vi "2 (1).vi"() -> ()   [LabVIEW 2015]
uses:
  <vilib>/NXT/Block Support/NXT_InputPort.ctl
  <vilib>/NXT/Block Support/NXT_OutputPort.ctl
  <vilib>/NXT/Dual Mode Library/Sensors/Sonar_cm.vi
  <vilib>/NXT/NXTIO Xnodes/NXTIONodeSubVIs/NXTMoveMotors.vi
  <vilib>/NXT/Dual Mode Library/Waits/Wait_Num.vi
  <vilib>/NXT/NXTIO Xnodes/AddressXNode/NXTIOAddress.xnode
  <vilib>/NXT/Subs/LVHSConnector.ctl
  <vilib>/NXT/NXTIO Xnodes/NXTIOXNode/NXTIO.xnode
  <vilib>/NXT/LegoClasses/BrickReference/BrickReference.lvclass
panel:
  in  "Power/Speed 4":i8=75
  in  "Power/Speed 3":i8=75
  in  "Time (1 sec) 2":sgl=1.0
  in  "Time (1 sec)":sgl=1.0
  in  "Power/Speed 1":i8=75
  in  "Port (Port 4)":T1=3 items=["Port 1", "Port 2", "Port 3", "Port 4"]
  in  "stop":bool
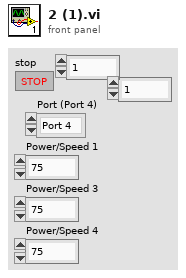
[diagram p1: front panel]
types:
  T1 = typedef "NXT_InputPort.ctl" = u32
  T2 = typedef "NXT_OutputPort.ctl" = u8
  T3 = cluster{"Output Port":T2, "Output Port 2":T2, "Output Port 3":T2}
  T4 = typedef "LVHSConnector.ctl" = refnum<class "BrickReference.lvclass">
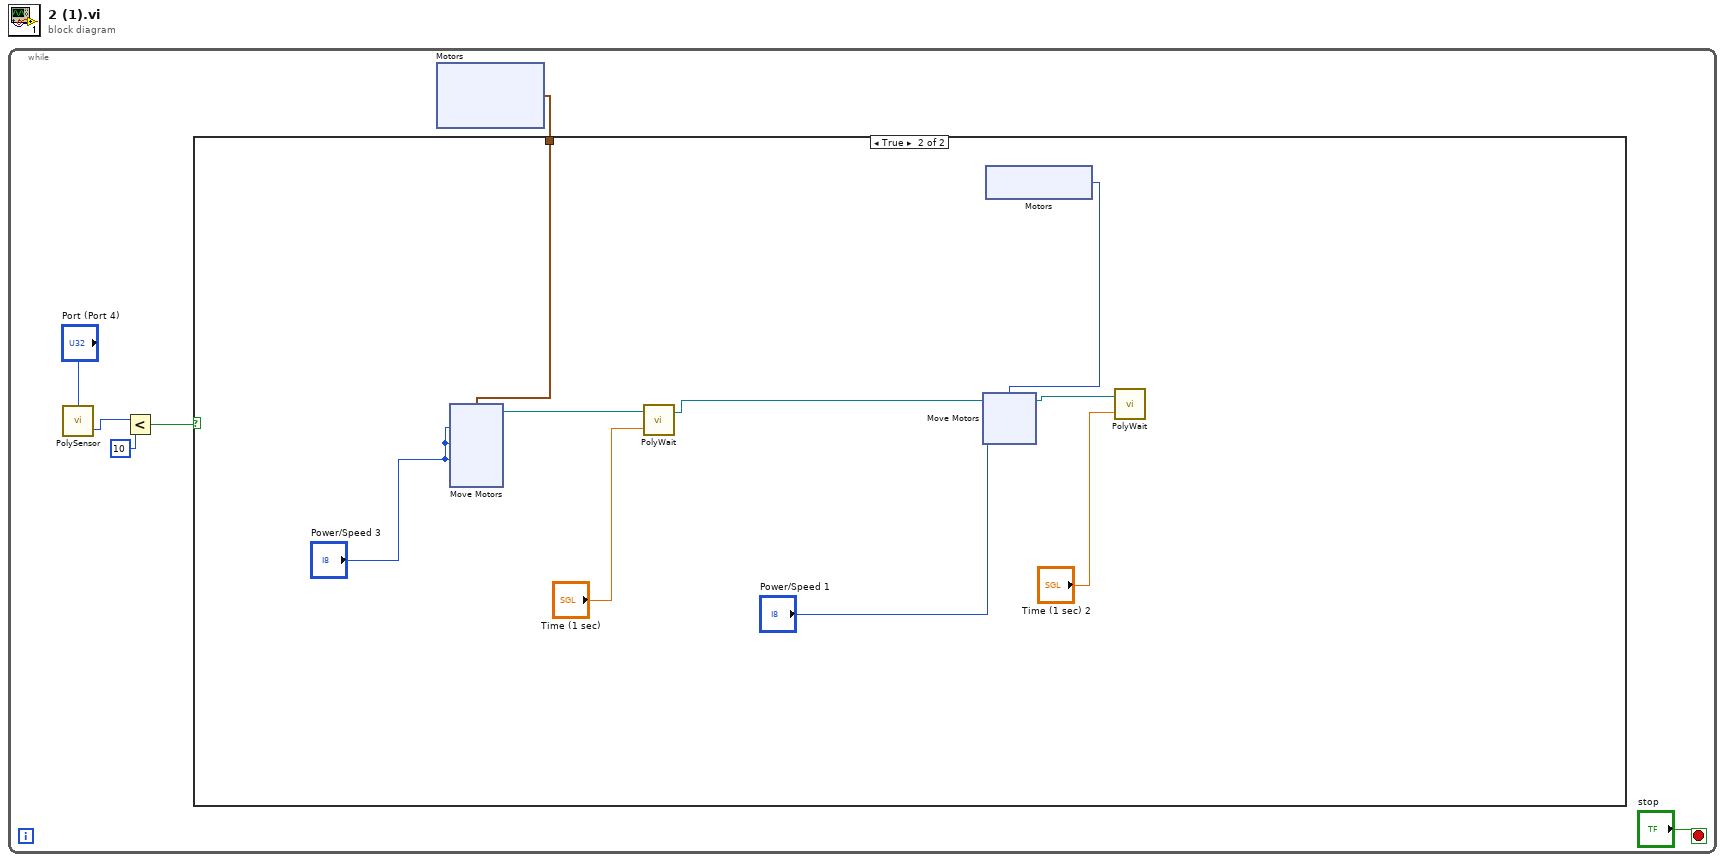
[diagram p0: block diagram]
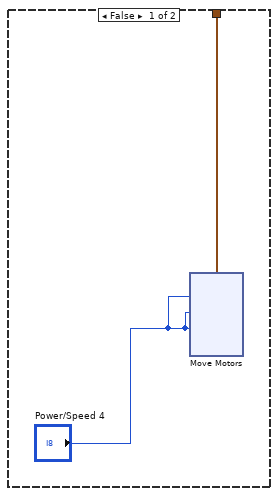
[diagram p2: hidden frame]
diagram:
  n1 = while {
    stop <- "stop" stop-if-true
    n2 = call-poly <vilib>:"PolySensor.vi"("Port (Port 4)"="Port (Port 4)") -> ("Distance (cm)"=w6:i16)  [unwired: 2 in, 1 out]
    n3 = Less?(x=w6, y=i16 10) -> (x < y?=w5:bool)
    n4 = xnode "Motors"() -> ("Motor"=w1:cluster{"Port":T2, "Port":T2, "Port":T2})
    n5 = case shown="True" w5 {
      tunnel: w1 -> [w9 w24]
      frame False {
        n6 = xnode "Move Motors"("Power/Speed 3"="Power/Speed 4", "Power/Speed 2"="Power/Speed 4", "Power/Speed 1"="Power/Speed 4", "Motors"=w9) -> ()  [unwired: 1 in, 1 out]
      }
      frame True {
        n7 = xnode "Move Motors"("Power/Speed 3"="Power/Speed 3", "Power/Speed 2"="Power/Speed 3", "Power/Speed 1"="Power/Speed 3", "Motors"=w24) -> ("NXT/EV3"=w27:T4)  [unwired: 1 in]
        n8 = call-poly <vilib>:"PolyWait.vi"("Time (1 sec)"="Time (1 sec)", "NXT/EV3"=w27) -> ("NXT/EV3"=w26:T4)  [unwired: 2 in]
        n9 = xnode "Motors"() -> ("Motor"=w23:T2)
        n10 = xnode "Move Motors"("Power/Speed 1"="Power/Speed 1", "Motors"=w23, "NXT/EV3"=w26) -> ("NXT/EV3"=w25:T4)
        n11 = call-poly <vilib>:"PolyWait.vi"("Time (1 sec)"="Time (1 sec) 2", "NXT/EV3"=w25) -> ()  [unwired: 2 in, 1 out]
      }
    }
  }
